vi "one_channel_send_wait_read.vi"() -> ()   [LabVIEW 2022 SP3]
uses:
  <instrlib>/Tektronix DPO MSO 2000 4000 Series/Public/Configure/Configure Trigger (Edge).vi
  <instrlib>/Tektronix DPO MSO 2000 4000 Series/Public/Data/Read (Single Waveform).vi
  <instrlib>/Tektronix DPO MSO 2000 4000 Series/Tektronix DPO MSO 2000 4000 Series.lvlib
  <instrlib>/Tektronix AFG 3000 Series/Tektronix AFG 3000 Series.lvlib
panel:
  in  "Enable Saving":bool
  in  "Filename":path=path "test.xlsx"
  in  "Vertical Range (100 mV)":dbl=10.0
  in  "Record Length (10: 10k points)":u32(ring)=10 items=["1000 points"=1, "10k points"=10, "100k points"=100, "1M points"=1000, "10M points"=10000]
  in  "Timebase (s)":dbl=4e-05
  in  "Trigger Channel":u16(ring) items=["Channel 1", "Channel 2", "Channel 3", "Channel 4", "Math", "Reference 1", "Reference 2", "Reference 3", "Reference 4"]
  in  "Trigger Level (V)":dbl
  in  "Enable Output":bool=TRUE
  in  "DC Offset (0.00 V)":dbl
  in  "Amplitude (1 Vpp)":dbl=1.0
  in  "Waveform Function (0: Sine)":u16(ring) items=["Sine", "Square", "Pulse", "Ramp", "Noise", "DC", "Sin(x)/x", "Gaussian", "Lorentz", "Exponential Rise", "Exponential Decay", "Haversine"]
  in  "Frequency (Hz)":dbl=1000.0
  in  "Burst Mode (0: Triggered)":u16(ring) items=["Triggered", "Gated"]
  in  "FN Wave Channel":u16(ring) items=["Channel 1", "Channel 2"]
  in  "Internal Trigger Rate (period in s)":dbl=500.0
  in  "Burst Count (5)":i32=5
  in  "FN Generator Name":refnum<visa-resource-name>
  in  "Listen Channel (0: Channel 1)":u16(ring) items=["Channel 1", "Channel 2", "Channel 3", "Channel 4", "Math", "Reference 1", "Reference 2", "Reference 3", "Reference 4"]
  in  "Maximum Time (ms)":u32=10000
  out "Waveform Graph":waveform(dbl)(graph)
  in  "Oscilloscope Name":refnum<visa-resource-name>
  # "File Controls"
  # "FN Generator Controls"
  # "Oscilloscope Controls"
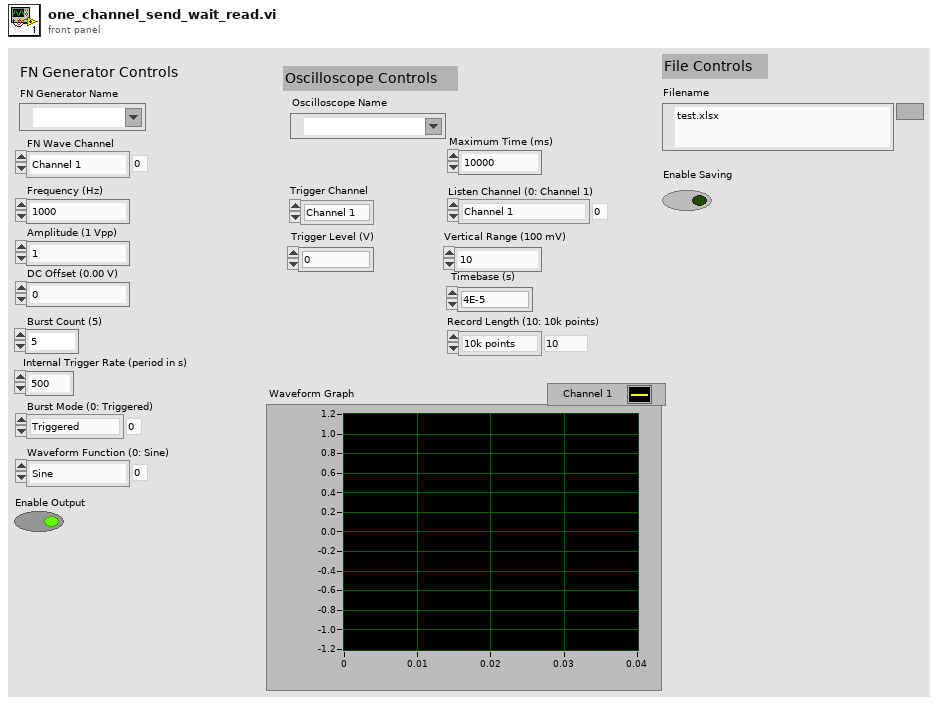
[diagram p1: front panel]
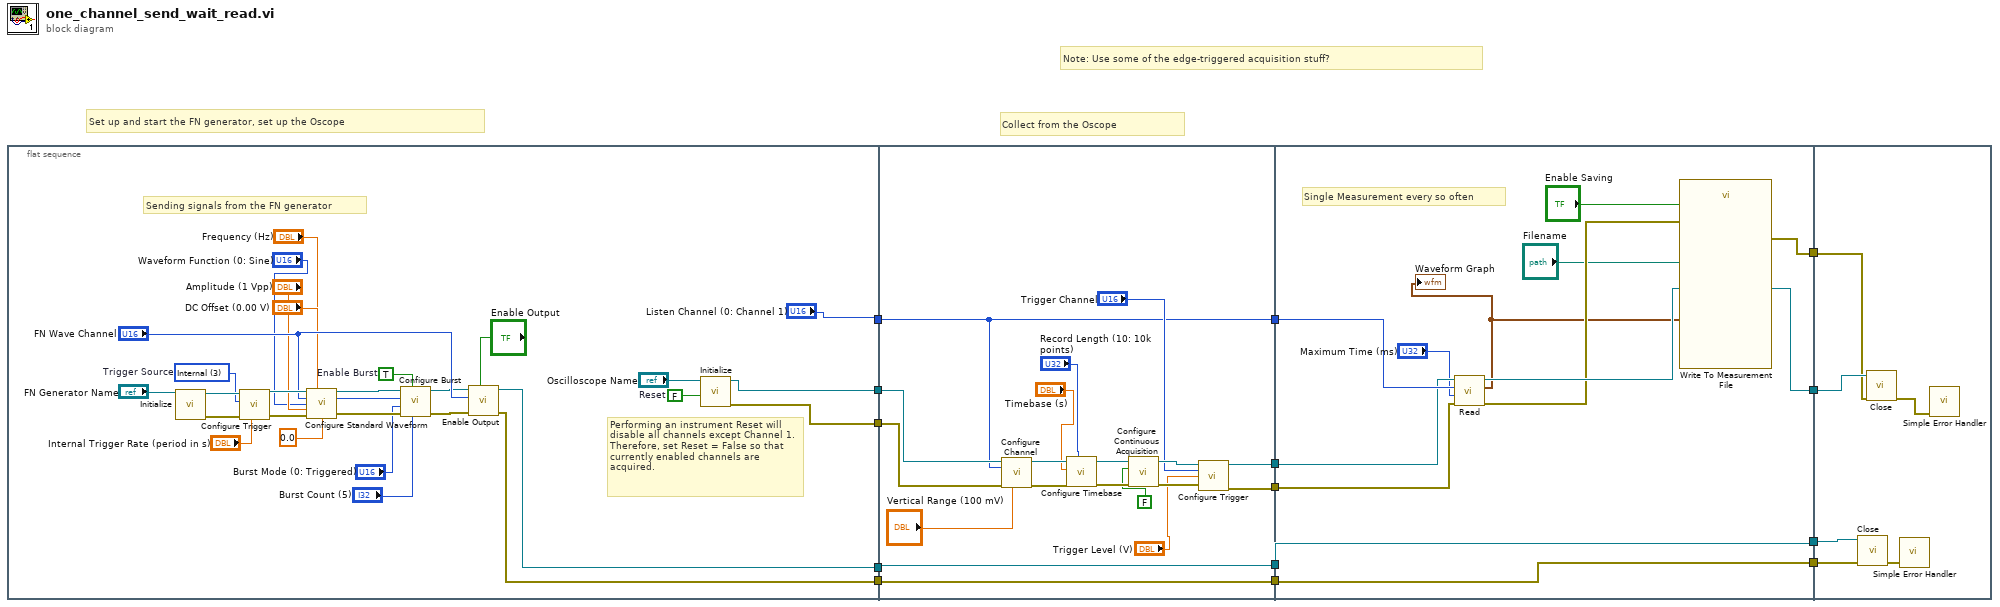
[diagram p0: block diagram]
diagram:
  # "Note: Use some of the edge-triggered acquisition stuff?"
  # "Collect from the Oscope"
  # "Set up and start the FN generator, set up the Oscope"
  n1 = flat-sequence {
    tunnel: ["Listen Channel (0: Channel 1)"] -> w11
    tunnel: [w18] -> w9
    tunnel: [w17] -> w7
    tunnel: [w16] -> w5
    tunnel: [w15] -> w4
    tunnel: w11 -> [w44]
    tunnel: [w44] -> w10
    tunnel: w9 -> [w61]
    tunnel: [w61] -> w8
    tunnel: w7 -> [w60]
    tunnel: [w60] -> w6
    tunnel: w5 -> [w56]
    tunnel: w4 -> [w57]
    tunnel: [w51] -> w3
    tunnel: [w49] -> w2
    tunnel: w10 -> [w71]
    tunnel: w8 -> [w73]
    tunnel: w6 -> [w72]
    tunnel: [w73] -> w14
    tunnel: [w72] -> w13
    tunnel: [w70] -> w12
    tunnel: w3 -> [w69]
    tunnel: w2 -> [w68]
    tunnel: [w64] -> w1
    tunnel: w14 -> [w78]
    tunnel: w13 -> [w77]
    tunnel: w12 -> [w75]
    tunnel: w1 -> [w74]
    frame #0 {
      w20 = FALSE  # Reset
      w23 = u16 3 items=["Internal"=3, "External"=1]  # Trigger Source
      w22 = TRUE  # Enable Burst
      # "Performing an instrument Reset will disable all channels except Channel 1. Therefore, set Reset = False so that currently enabled channels are acquired."
      # "Sending signals from the FN generator"
      n2 = call <instrlib>:"Initialize.vi"("VISA resource name"="FN Generator Name") -> ("error out"=w31:errorcluster, "VISA resource name out"=w30:refnum<visa-resource-name>)  [unwired: 9 in]
      n3 = call <instrlib>:"Configure Trigger.vi"("Internal Trigger Rate (500)"="Internal Trigger Rate (period in s)", "error in (no error)"=w31, "Trigger Source (3:Internal)"=w23, "VISA resource name"=w30) -> ("error out"=w41:errorcluster, "VISA resource name out"=w38:refnum<visa-resource-name>)  [unwired: 6 in]
      n4 = call <instrlib>:"Configure Standard Waveform.vi"("VISA resource name"=w38, "Frequency (1000 Hz)"="Frequency (Hz)", "Channel (0: Channel 1)"="FN Wave Channel", "Waveform Function (0: Sine)"="Waveform Function (0: Sine)", "Amplitude (1 Vpp)"="Amplitude (1 Vpp)", "error in (no error)"=w41, "DC Offset (0.00 V)"="DC Offset (0.00 V)", "Phase Level (-1)"=0.0) -> ("VISA resource name out"=w39:refnum<visa-resource-name>, "error out"=w42:errorcluster)  [unwired: 6 in]
      n5 = call <instrlib>:"Configure Burst.vi"("Burst Count (5)"="Burst Count (5)", "Enable Burst (T: Enable)"=w22, "error in (no error)"=w42, "Burst Mode (0: Triggered)"="Burst Mode (0: Triggered)", "Channel (0: Channel 1)"="FN Wave Channel", "VISA resource name"=w39) -> ("error out"=w26:errorcluster, "VISA resource name out"=w25:refnum<visa-resource-name>)  [unwired: 4 in]
      n6 = call <instrlib>:"Enable Output.vi"("Enable Output (T: Enable)"="Enable Output", "error in (no error)"=w26, "Channel (0: Channel 1)"="FN Wave Channel", "VISA resource name"=w25) -> ("error out"=w18:errorcluster, "VISA resource name out"=w17:refnum<visa-resource-name>)  [unwired: 6 in]
      n7 = call <instrlib>:"Initialize.vi"("Reset (True)"=w20, "VISA resource name"="Oscilloscope Name") -> ("error out"=w16:errorcluster, "VISA resource name out"=w15:refnum<visa-resource-name>)  [unwired: 8 in]
    }
    frame #1 {
      n8 = call <instrlib>:"Configure Channel.vi"("VISA resource name"=w57, "Channel (0: Channel 1)"=w44, "error in (no error)"=w56, "Vertical Range (10.0 V)"="Vertical Range (100 mV)") -> ("VISA resource name out"=w59:refnum<visa-resource-name>, "error out"=w55:errorcluster)  [unwired: 10 in]
      n9 = call <instrlib>:"Configure Timebase.vi"("Record Length (10: 10k points)"="Record Length (10: 10k points)", "error in (no error)"=w55, "Timebase (0.0005 s)"="Timebase (s)", "VISA resource name"=w59) -> ("error out"=w54:errorcluster, "VISA resource name out"=w58:refnum<visa-resource-name>)  [unwired: 6 in]
      n10 = call <instrlib>:"Configure Continuous Acquisition.vi"("error in (no error)"=w54, "Enable Continuous Acquisition Mode (T: Enable)"=FALSE, "VISA resource name"=w58) -> ("error out"=w50:errorcluster, "VISA resource name out"=w52:refnum<visa-resource-name>)  [unwired: 7 in]
      n11 = call-poly <instrlib>:"Configure Trigger.vi"("VISA resource name"=w52, "Trigger Source (0: Channel 1)"="Trigger Channel", "Trigger Level (0.0 V)"="Trigger Level (V)", "error in (no error)"=w50) -> ("VISA resource name out"=w51:refnum<visa-resource-name>, "error out"=w49:errorcluster)  [unwired: 10 in]
    }
    frame #2 {
      # "Single Measurement every so often"
      n12 = call-poly <instrlib>:"Read.vi"("error in (no error)"=w68, "Maximum Time (10000ms)"="Maximum Time (ms)", "Channel (0: Channel 1)"=w71, "VISA resource name"=w69) -> ("error out"=w66:errorcluster, "Waveform Graph"=w65:waveform(dbl), "VISA resource name out"=w70:refnum<visa-resource-name>)  [unwired: 5 in]
      "Waveform Graph" <- w65
      n13 = call "Write To Measurement File"("Signals"=w65, "Enable"="Enable Saving", "error in (no error)"=w66, "Filename"="Filename") -> ("error out"=w64:errorcluster)  [unwired: 13 in, 2 out]
    }
    frame #3 {
      n14 = call <instrlib>:"Close.vi"("error in (no error)"=w78, "VISA resource name"=w77) -> ("error out"=w79:errorcluster)  [unwired: 9 in]
      n15 = call <instrlib>:"Close.vi"("error in (no error)"=w74, "VISA resource name"=w75) -> ("error out"=w76:errorcluster)  [unwired: 9 in]
      n16 = call <vilib>:"Simple Error Handler.vi"("error in (no error)"=w79) -> ()  [unwired: 4 in, 5 out]
      n17 = call <vilib>:"Simple Error Handler.vi"("error in (no error)"=w76) -> ()  [unwired: 4 in, 5 out]
    }
  }
